vi "main_project.vi"() -> ()   [LabVIEW 2021]
panel:
  out "out":T1(array[cluster])
  out "XML String":string
  in  "path_to_store":path
  out "output array":T2(array[cluster])
  in  "Tag":T3(ring)
  out "mouse_up":bool
  out "mouse_down":bool
  in  "image":path
  in  "stop":bool
  out "Image 2":T4(plugin-control)
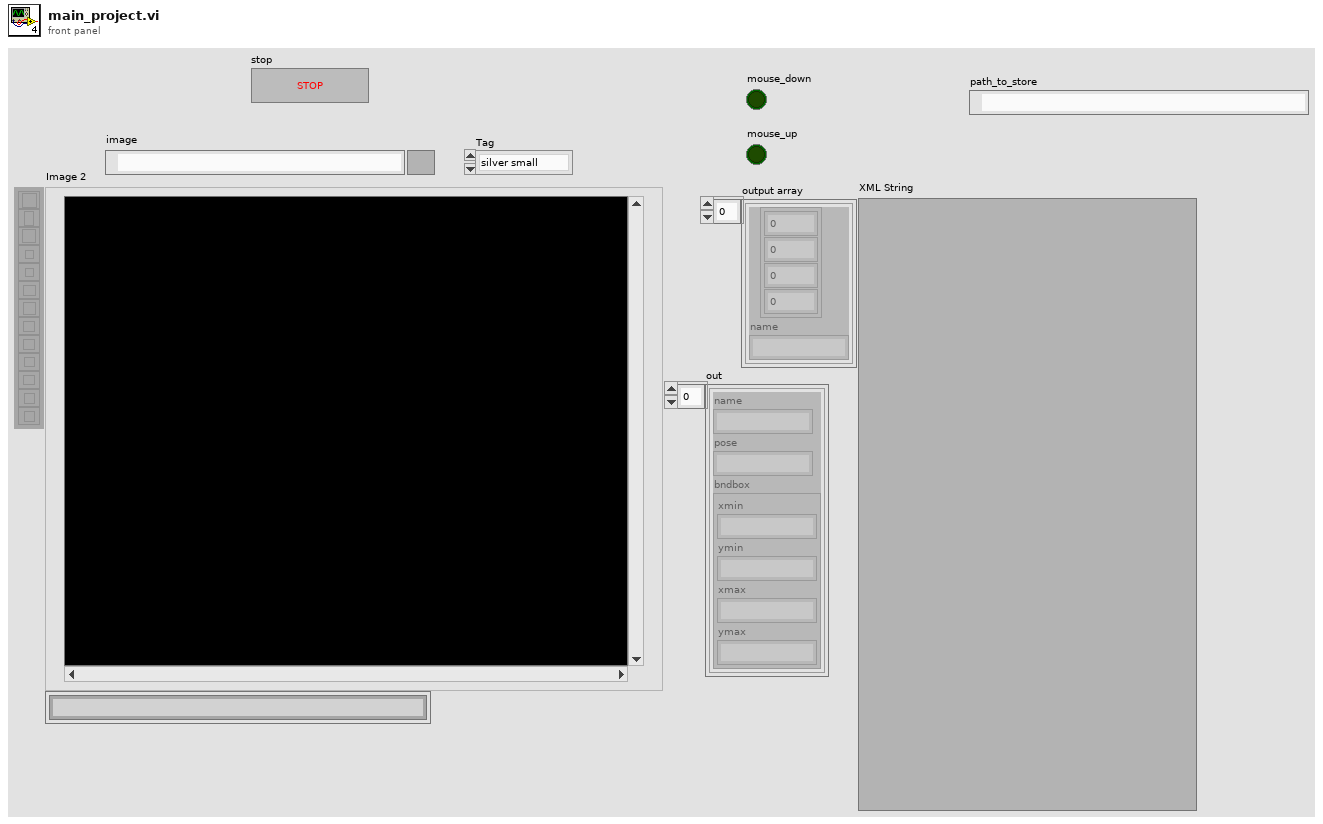
[diagram p1: front panel]
types:
  T1 = cluster{"name":string, "pose":string, "bndbox":cluster{"xmin":string, "ymin":string, "xmax ":string, "ymax":string}}[]
  T2 = cluster{cluster{i32, i32, i32, i32}, "name":string}[]
  T3 = enum16{"silver small", "silver medium", "silver huge", "black small", "black medium", "black huge"}
  T4 = typedef "IMAQ Image.ctl" = refnum<image>
  T5 = cluster{"width":string, "height":string, "depth ":string}
  T6 = cluster{"Global Rectangle":i32[], "Contours":cluster{"Contour Type":u32, "ROI Type":u32, "Points":i32[]}[]}
  T7 = cluster{cluster{i32, i32, i32, i32}, "name":string}
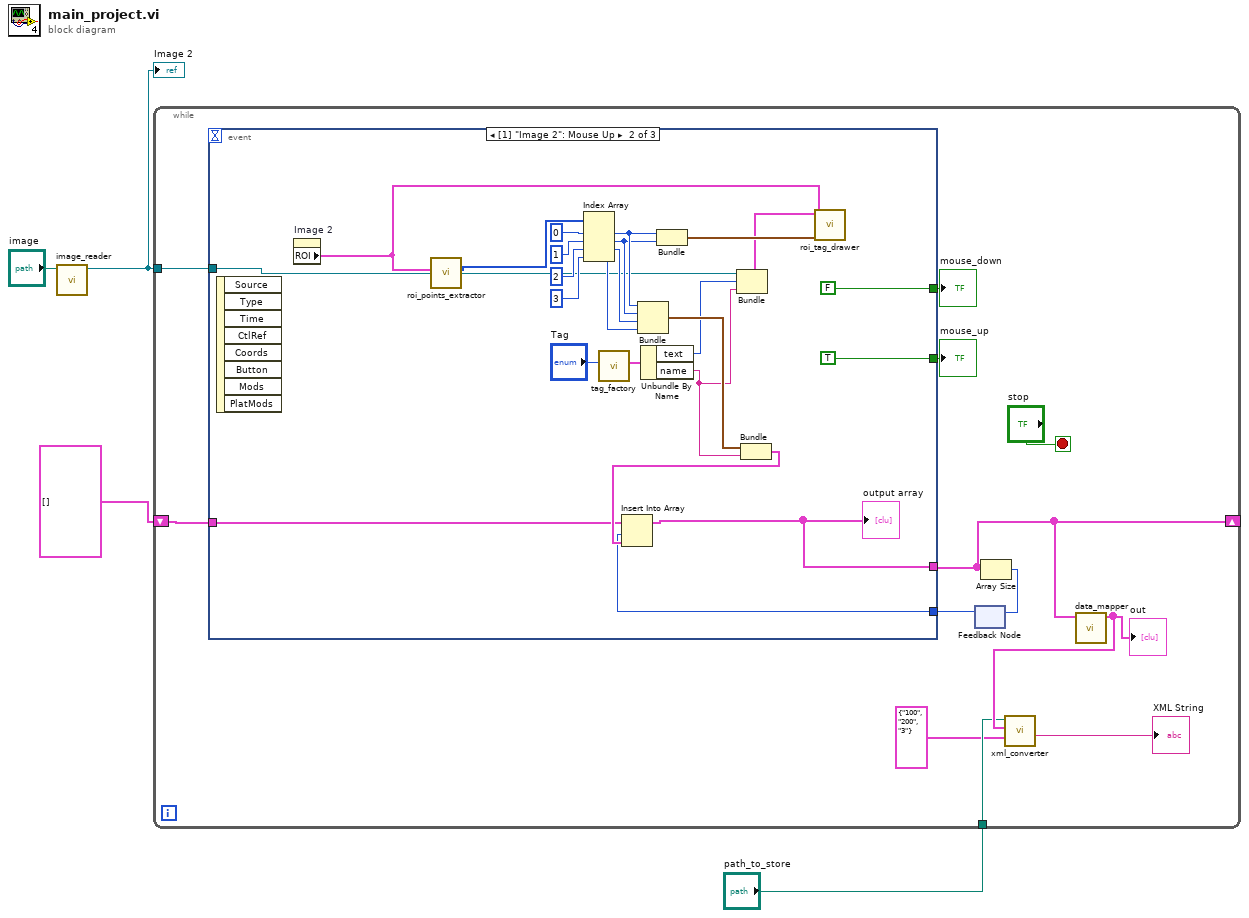
[diagram p0: block diagram]
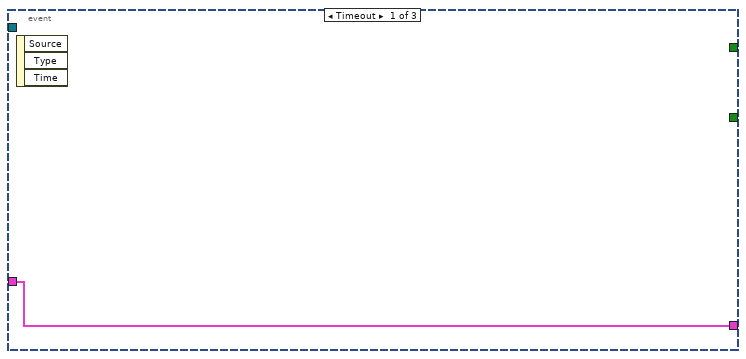
[diagram p2: hidden frame]
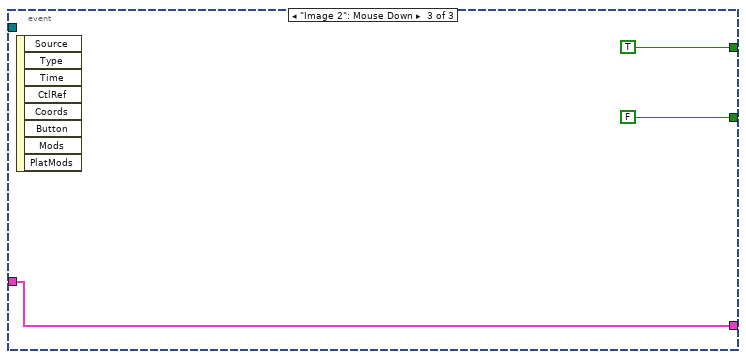
[diagram p3: hidden frame]
diagram:
  n1 = call "image_reader.vi"("input image 2"="image") -> ("Image 2"=w4:T4)  [unwired: 10 in]
  "Image 2" <- w4
  n2 = while {
    tunnel: w4 -> [w15]
    shift-right: [w9] -> _
    shift-left: T2 [] ("array") -> [w10]
    tunnel: "path_to_store" -> [w7]
    stop <- "stop" stop-if-true
    n3 = feedback #1() -> (w11:i32)  [unwired: 1 in]
    n4 = event shown="[1] \"Image 2\": Mouse Up" {
      selector: _ -> [_ _ _]
      dyn-events: _ -> [_ _ _]
      timeout: _ -> [_ _ _]
      tunnel: w15 -> [_ w19 _]
      tunnel: [_ FALSE TRUE] -> w14
      tunnel: [_ TRUE ("mouse_up") FALSE ("mouse_up")] -> w13
      tunnel: w10 -> [w17 w27 w42]
      tunnel: [w17 w26 w42] -> w9
      tunnel: w11 -> [_ w25 _]
      event Timeout {
        n5 = event-data() -> ()  [unwired: 1 in, 3 out]
      }
      event "Image 2": Mouse Up {
        n6 = event-data() -> ()  [unwired: 1 in, 8 out]
        n7 = property on="Image 2" class="ImageControl"() -> ("ROI"=w22:T6)  [unwired: 2 in, 2 out]
        n8 = call "roi_points_extractor.vi"("input cluster"=w22) -> ("Points"=w24:i32[])  [unwired: 10 in]
        n9 = Index Array(array=w24, index #1=0 ("index"), index #2=1 ("index"), index #3=2 ("index"), index #4=3 ("index")) -> (element #1=w33:i32, element #2=w32:i32, element #3=w31:i32, element #4=w30:i32)
        n10 = call "tag_factory.vi"("Enum"="Tag") -> ("Cluster"=w37:cluster{"name":string, "text":u32})  [unwired: 10 in]
        n11 = Bundle(w33, w32, w31, w30) -> (w29:cluster{i32, i32, i32, i32})  [unwired: 1 in]
        n12 = Unbundle By Name(w37) -> ("text"=w21:u32, "name"=w20:string)
        n13 = Bundle(w33, w32) -> (w23:cluster{i32, i32})  [unwired: 1 in]
        n14 = Bundle("Image 2"=w19, "text"=w21, "name"=w20) -> (w18:cluster{"Image 2":T4, "text":u32, "name":string})  [unwired: 1 in]
        n15 = Bundle(w29, "name"=w20) -> (w28:T7)  [unwired: 1 in]
        n16 = Insert Into Array(array=w27, index=w25, new element=w28) -> (w26:T2)
        "output array" <- w26
        n17 = call "roi_tag_drawer.vi"("Origin"=w23, "ROI Descriptor"=w22, "Cluster"=w18) -> ()  [unwired: 9 in]
      }
      event "Image 2": Mouse Down {
        n18 = event-data() -> ()  [unwired: 1 in, 8 out]
      }
    }
    "mouse_down" <- w14
    "mouse_up" <- w13
    n19 = Array Size(array=w9) -> (size(s)=w12:i32)
    n20 = feedback-in #1(w12) -> ()
    n21 = call "data_mapper.vi"("input"=w9) -> ("out"=w8:T1)  [unwired: 10 in]
    "out" <- w8
    n22 = call "xml_converter.vi"("size"=T5 {"width"="100", "height"="200", "depth "="3"}, "object"=w8, "XML File Path 2"=w7) -> ("XML String"=→"XML String":string)  [unwired: 4 in]
  }
